vi "Teleop Drivetrain Control.vi"(11 "Axes":T1) -> ()   [LabVIEW 2017]
uses:
  Common Code/Gamepads/Axes Cluster.ctl
  Robot Global Data.vi
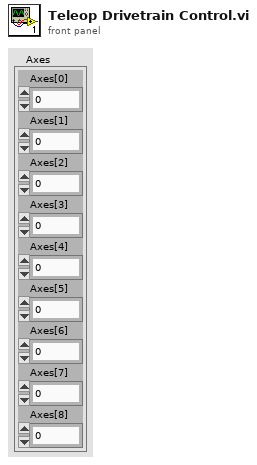
[diagram p1: front panel]
types:
  T1 = typedef "Axes Cluster.ctl" = cluster{"Axes[0]":dbl, "Axes[1]":dbl, "Axes[2]":dbl, "Axes[3]":dbl, "Axes[4]":dbl, "Axes[5]":dbl, "Axes[6]":dbl, "Axes[7]":dbl, "Axes[8]":dbl}
  T2 = typedef "Teleop Command Cluster.ctl" = cluster{"Y power":dbl, "Turn Power":dbl}
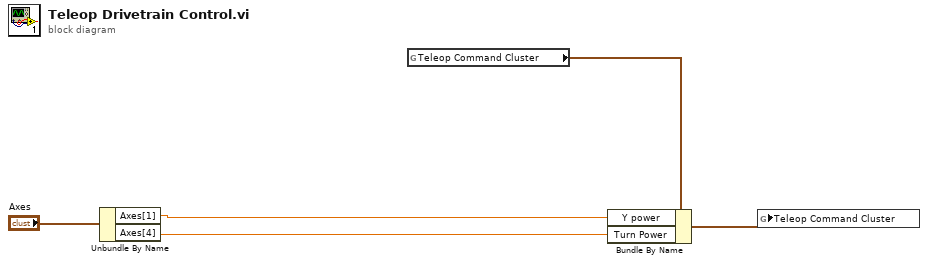
[diagram p0: block diagram]
diagram:
  n1 = Unbundle By Name("Axes") -> ("Axes[1]"=w2:dbl, "Axes[4]"=w1:dbl)
  n2 = global read "Robot Global Data.vi" "Teleop Command Cluster"() -> (w4:T2)
  n3 = Bundle By Name(cluster=w4, "Y power"=w2, "Turn Power"=w1) -> (w3:T2)
  n4 = global write "Robot Global Data.vi" "Teleop Command Cluster"(w3) -> ()
